vi "Remove final slash.vi"(11 "SVN":T1) -> (3 "SVN out":T1)   [LabVIEW 2012]
uses:
  SVN.ctl
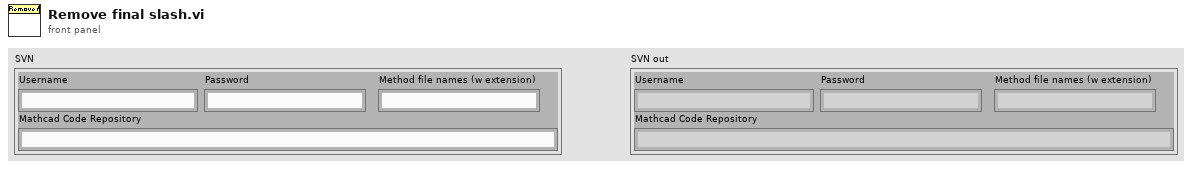
[diagram p1: front panel]
types:
  T1 = typedef "SVN.ctl" = cluster{"Mathcad Code Repository":string, "Username":string, "Password":string, "Method file names (w extension)":string}
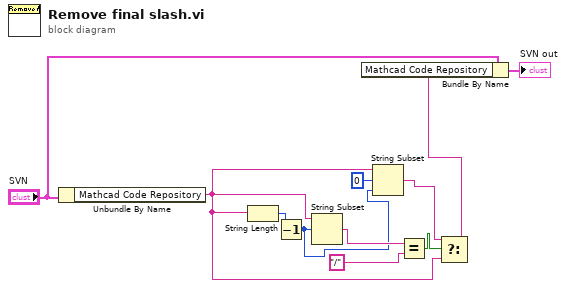
[diagram p0: block diagram]
diagram:
  n1 = Unbundle By Name("SVN") -> ("Mathcad Code Repository"=w4:string)
  n2 = String Length(string=w4) -> (length=w9:i32)
  n3 = Decrement(x=w9) -> (x-1=w2:i32)
  n4 = String Subset(string=w4, offset (0)=w2) -> (substring=w8:string)  [unwired: 1 in]
  n5 = String Subset(string=w4, offset (0)=0, length (rest)=w2) -> (substring=w1:string)
  n6 = Equal?(x=w8, y="/" ("substring")) -> (x = y?=w6:bool)
  n7 = Select(t=w1, s=w6, f=w4) -> (s? t:f=w5:string)
  n8 = Bundle By Name(cluster="SVN", "Mathcad Code Repository"=w5) -> (→"SVN out":T1)
